vi "Convert Array of Bytes to String (RX and TX).vi"(10 "RX_array":u8[][](array[numeric]), 11 "TX_array":u8[](array[numeric])) -> (2 "RX":string, 3 "TX":string)   [LabVIEW 2023]
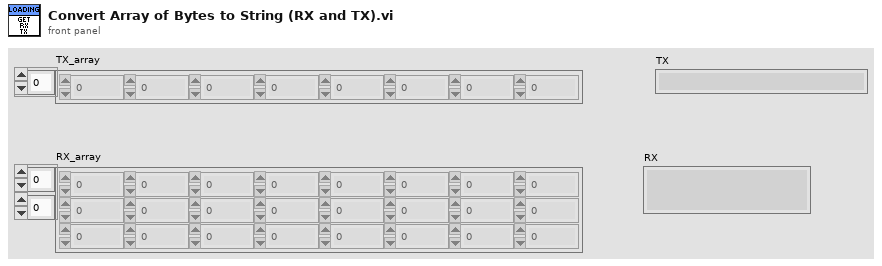
[diagram p1: front panel]
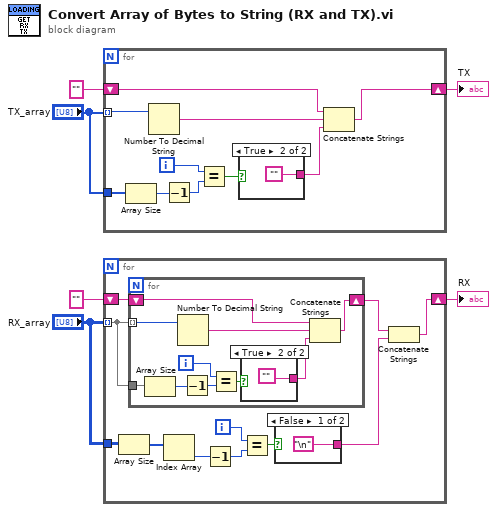
[diagram p0: block diagram]
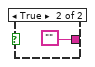
[diagram p2: hidden frame]
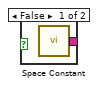
[diagram p3: hidden frame]
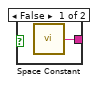
[diagram p4: hidden frame]
diagram:
  n1 = for {
    tunnel: "TX_array" -> [w12] mode=indexing
    shift-right: [w14] -> w5
    shift-left: "" -> [w13]
    tunnel: "TX_array" -> [w11]
    i -> [w8]
    n2 = Array Size(array=w11) -> (size(s)=w10:i32)
    n3 = Number To Decimal String(number=w12) -> (decimal integer string=w16:string)  [unwired: 1 in]
    n4 = Decrement(x=w10) -> (x-1=w9:i32)
    n5 = Equal?(x=w8, y=w9) -> (x = y?=w7:bool)
    n6 = case shown="True" w7 {
      tunnel: [w17 "" ("String")] -> w15
      frame False {
        n7 = call <vilib>:"Space Constant.vi"() -> ("String"=w17:string)
      }
      frame True {
      }
    }
    n8 = Concatenate Strings(w13, w16, w15) -> (w14:string)
  }
  "TX" <- w5
  n9 = for {
    tunnel: "RX_array" -> [w19] mode=indexing
    shift-right: [w27] -> w3
    shift-left: "" -> [w29]
    tunnel: "RX_array" -> [w25]
    i -> [w21]
    n10 = Array Size(array=w25) -> (size(s)=w24:i32[])
    n11 = for {
      tunnel: w19 -> [w36] mode=indexing
      shift-right: [w39] -> w28
      shift-left: w29 -> [w40]
      tunnel: w19 -> [w35]
      i -> [w33]
      n12 = Array Size(array=w35) -> (size(s)=w37:i32)
      n13 = Number To Decimal String(number=w36) -> (decimal integer string=w41:string)  [unwired: 1 in]
      n14 = Decrement(x=w37) -> (x-1=w34:i32)
      n15 = Equal?(x=w33, y=w34) -> (x = y?=w32:bool)
      n16 = case shown="True" w32 {
        tunnel: [w42 "" ("String")] -> w38
        frame False {
          n17 = call <vilib>:"Space Constant.vi"() -> ("String"=w42:string)
        }
        frame True {
        }
      }
      n18 = Concatenate Strings(w40, w41, w38) -> (w39:string)
    }
    n19 = Index Array(array=w24) -> (element=w23:i32)  [unwired: 1 in]
    n20 = Decrement(x=w23) -> (x-1=w22:i32)
    n21 = Equal?(x=w21, y=w22) -> (x = y?=w20:bool)
    n22 = case shown="False" w20 {
      tunnel: ["\n" ("string") "" ("String")] -> w26
      frame False {
      }
      frame True {
      }
    }
    n23 = Concatenate Strings(w28, w26) -> (w27:string)
  }
  "RX" <- w3
